vi "8.5.vi"() -> ()   [LabVIEW 2017]
panel:
  out "wortel":dbl
  in  "x":dbl
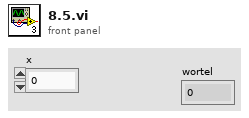
[diagram p1: front panel]
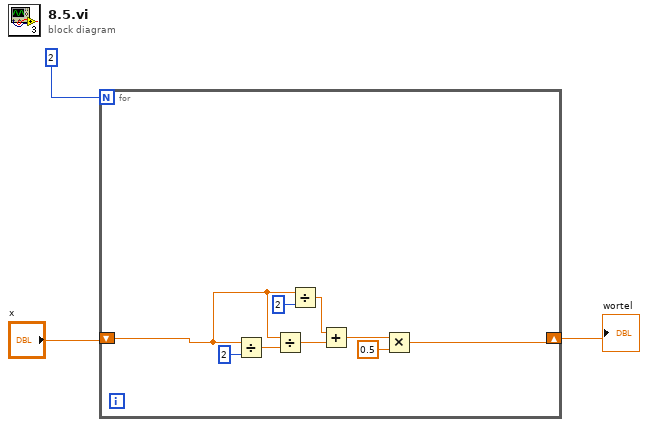
[diagram p0: block diagram]
diagram:
  n1 = for {
    N: 2 -> [_]
    shift-right: [w4] -> w2
    shift-left: "x" -> [w5]
    n2 = Divide(x=w5, y=2) -> (x/y=w9:dbl)
    n3 = Divide(x=w5, y=w9) -> (x/y=w11:dbl)
    n4 = Divide(x=w5, y=2) -> (x/y=w10:dbl)
    n5 = Add(x=w10, y=w11) -> (x+y=w12:dbl)
    n6 = Multiply(x=w12, y=0.5) -> (x*y=w4:dbl)
  }
  "wortel" <- w2
